vi "ExSubStripFlag.vi"(0 "Binning \nUser = 1\nCenter = 2\nFull = 3":u32=1 min=1 max=3 step=1) -> ()   [LabVIEW 2010]
uses:
  Spectroscopy Applications/GlobalCenter.vi
  GlobalFullBin.vi
  GlobalUserBin.vi
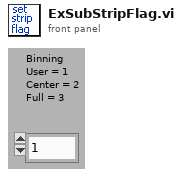
[diagram p1: front panel]
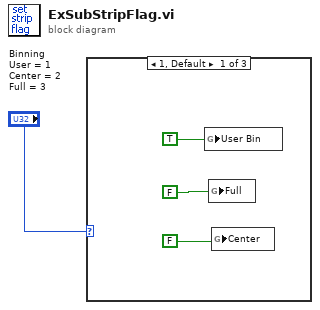
[diagram p0: block diagram]
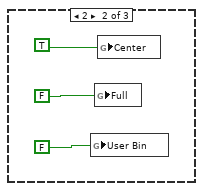
[diagram p2: hidden frame]
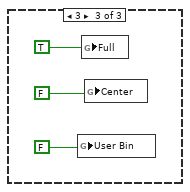
[diagram p3: hidden frame]
diagram:
  n1 = case shown="1, Default" "Binning \nUser = 1\nCenter = 2\nFull = 3" {
    frame 1, Default {
      n2 = global write "GlobalUserBin.vi" "User Bin"(TRUE) -> ()
      n3 = global write "GlobalFullBin.vi" "Full"(FALSE) -> ()
      n4 = global write "GlobalCenter.vi" "Center"(FALSE) -> ()
    }
    frame 2 {
      n5 = global write "GlobalUserBin.vi" "User Bin"(FALSE) -> ()
      n6 = global write "GlobalFullBin.vi" "Full"(FALSE) -> ()
      n7 = global write "GlobalCenter.vi" "Center"(TRUE) -> ()
    }
    frame 3 {
      n8 = global write "GlobalUserBin.vi" "User Bin"(FALSE) -> ()
      n9 = global write "GlobalFullBin.vi" "Full"(TRUE) -> ()
      n10 = global write "GlobalCenter.vi" "Center"(FALSE) -> ()
    }
  }
